vi "ellipse.vi"() -> ()   [LabVIEW 2020]
panel:
  out "XY Graph":cluster{dbl[], dbl[]}[](graph)
  in  "Major B":dbl
  in  "Major Axis A":dbl
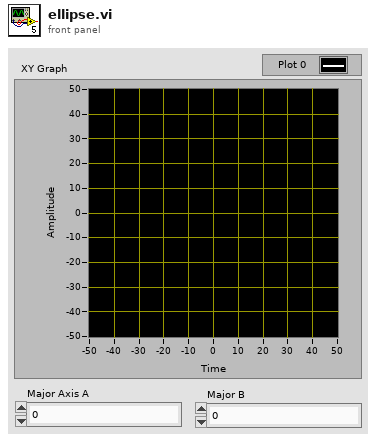
[diagram p1: front panel]
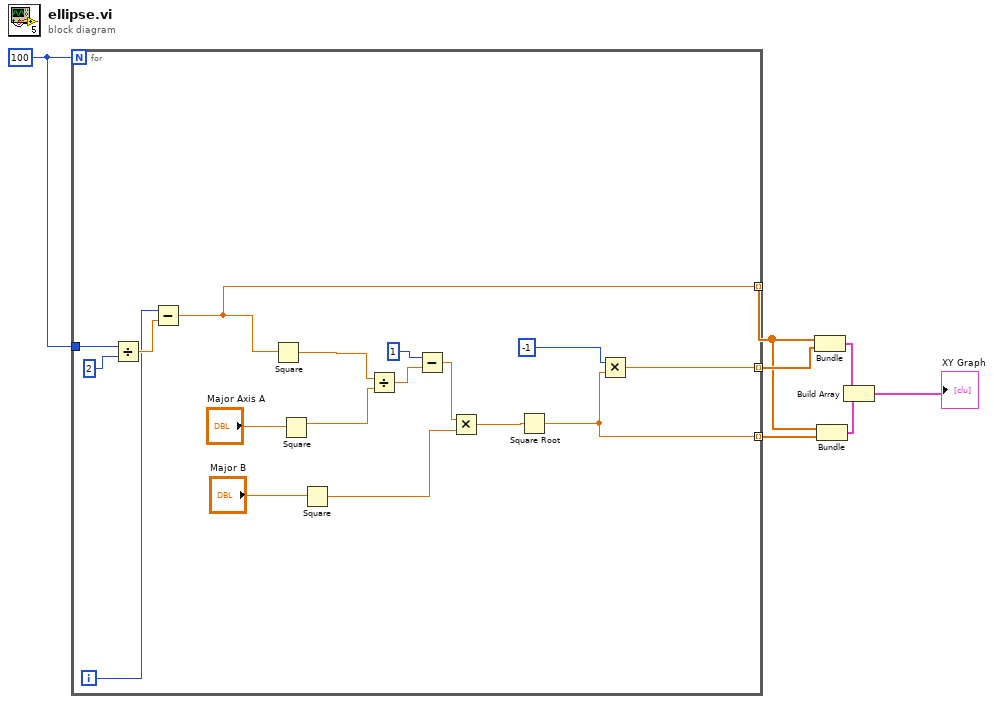
[diagram p0: block diagram]
diagram:
  w1 = 100
  n1 = for {
    N: w1 -> [_]
    tunnel: [w8] -> w5 mode=indexing
    tunnel: [w14] -> w7 mode=indexing
    tunnel: [w13] -> w6 mode=indexing
    tunnel: w1 -> [w11]
    i -> [w9]
    n2 = Divide(x=w11, y=2) -> (x/y=w10:dbl)
    n3 = Subtract(x=w9, y=w10) -> (x-y=w8:dbl)
    n4 = Square(x=w8) -> (x^2=w21:dbl)
    n5 = Square(x="Major Axis A") -> (x^2=w22:dbl)
    n6 = Square(x="Major B") -> (x^2=w17:dbl)
    n7 = Divide(x=w21, y=w22) -> (x/y=w19:dbl)
    n8 = Subtract(x=1, y=w19) -> (x-y=w18:dbl)
    n9 = Multiply(x=w18, y=w17) -> (x*y=w16:dbl)
    n10 = Square Root(x=w16) -> (sqrt(x)=w14:dbl)
    n11 = Multiply(x=-1, y=w14) -> (x*y=w13:dbl)
  }
  n12 = Bundle(w5, w6) -> (w4:cluster{dbl[], dbl[]})  [unwired: 1 in]
  n13 = Bundle(w5, w7) -> (w3:cluster{dbl[], dbl[]})  [unwired: 1 in]
  n14 = Build Array(w4, w3) -> (→"XY Graph":cluster{dbl[], dbl[]}[])
